vi "split_text_to_nodes.vi"(7 "max_character_length":u32, 10 "metadatas":cluster{"key":string, "value":string}[](array[cluster]), 11 "text":string) -> (3 "Nodes":refnum<class "data_node.lvclass">[](array[class]))   [LabVIEW 2020, in "chunk_character_splitter.lvclass"]
uses:
  chunk_character_splitter.lvclass
  data/data_node/data_node.lvclass
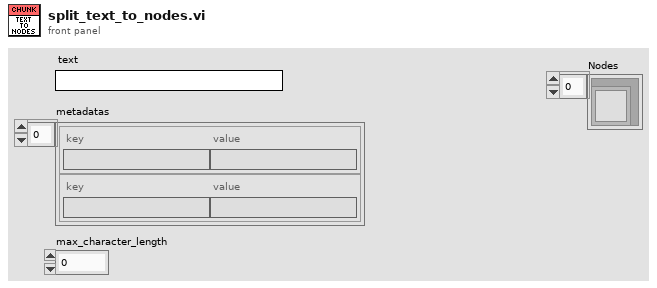
[diagram p1: front panel]
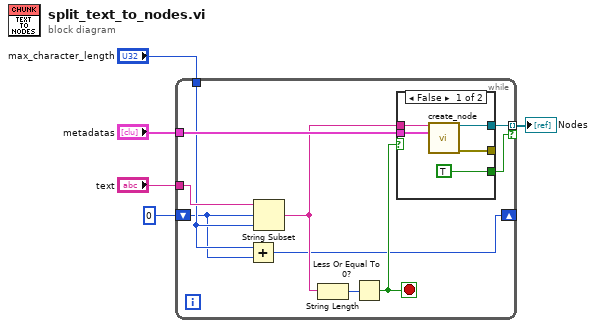
[diagram p0: block diagram]
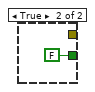
[diagram p2: hidden frame]
diagram:
  n1 = while {
    tunnel: "metadatas" -> [w14]
    tunnel: "max_character_length" -> [w8]
    shift-right: [w6] -> _
    shift-left: 0 -> [w7]
    tunnel: "text" -> [w15]
    tunnel: [w13] -> w1 mode=indexing if=w9
    stop <- w10 stop-if-true
    n2 = Add(x=w8, y=w7) -> (x+y=w6:u32)
    n3 = String Subset(string=w15, offset (0)=w7, length (rest)=w8) -> (substring=w12:string)
    n4 = String Length(string=w12) -> (length=w11:i32)
    n5 = Less Or Equal To 0?(x=w11) -> (x <= 0?=w10:bool)
    n6 = case shown="False" w10 {
      tunnel: w14 -> [w20 _]
      tunnel: [w19 _] -> w13
      tunnel: w12 -> [w18 _]
      tunnel: [TRUE FALSE] -> w9
      tunnel: [w16 _] -> _
      frame False {
        n7 = call "create_node.vi"("text"=w18, "metadatas"=w20) -> ("data_node out"=w19:refnum<class "data_node.lvclass">, "error out"=w16:errorcluster)  [unwired: 12 in]
      }
      frame True {
      }
    }
  }
  "Nodes" <- w1
